vi "储存测试.vi"() -> ()   [LabVIEW 2019, in "test.lvlib"]
uses:
  SubVI/test.lvlib
  <vilib>/Utility/file.llb/Write Delimited Spreadsheet (I64).vi
panel:
  in  "名称或相对路径":string
  out "添加的路径":path
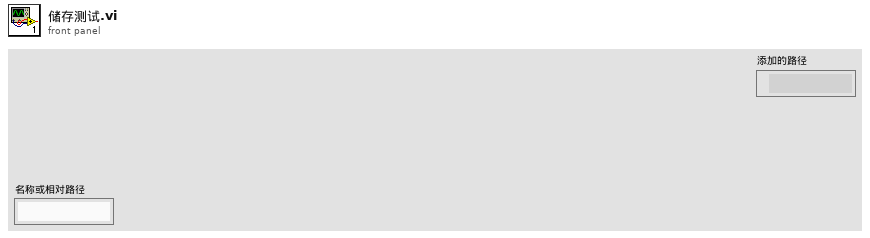
[diagram p1: front panel]
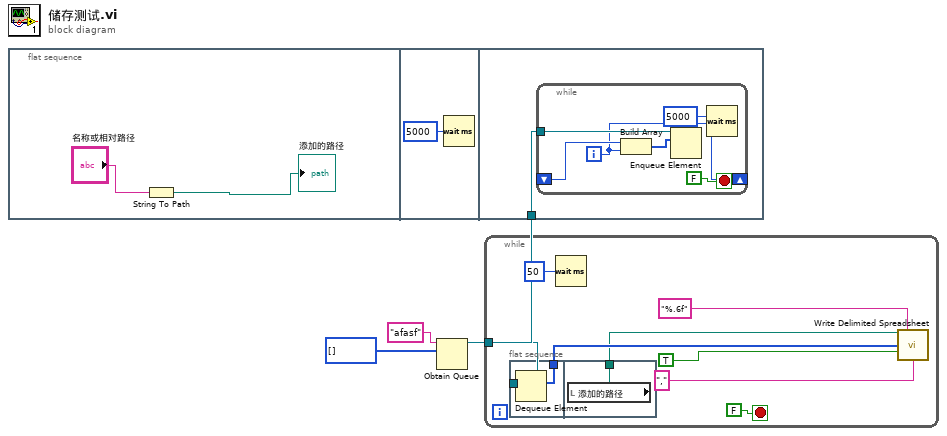
[diagram p0: block diagram]
diagram:
  n1 = flat-sequence {
    tunnel: w1 -> [w7]
    frame #0 {
      n2 = String To Path(string="名称或相对路径") -> (path=→"添加的路径":path)
    }
    frame #1 {
      n3 = Wait (ms)(milliseconds to wait=u32 5000 ("等待时间（毫秒）")) -> ()  [unwired: 1 out]
    }
    frame #2 {
      n4 = while {
        tunnel: w7 -> [w13]
        shift-right: [w11] -> _
        shift-left: _ -> [w12]
        i -> [w11]
        stop <- FALSE stop-if-true
        n5 = Build Array(w12, w11) -> (w10:i32[])
        n6 = Enqueue Element(queue=w13, element=w10) -> ()  [unwired: 2 in, 3 out]
        n7 = Wait (ms)(milliseconds to wait=u32 5000 ("等待时间（毫秒）")) -> ()  [unwired: 1 out]
      }
    }
  }
  n8 = Obtain Queue(name (unnamed)="afasf" ("名称（未命名）"), element data type=i32[] []) -> (queue out=w1:refnum<queue>)  [unwired: 3 in, 2 out]
  n9 = while {
    tunnel: w1 -> [w16]
    stop <- FALSE stop-if-true
    n10 = flat-sequence {
      tunnel: w16 -> [w23]
      tunnel: [w22] -> w15
      tunnel: [w24] -> w14
      frame #0 {
        n11 = Dequeue Element(queue=w23) -> (element=w22:i32[])  [unwired: 2 in, 3 out]
      }
      frame #1 {
        n12 = local read "添加的路径"() -> (w24:path)
      }
    }
    n13 = Wait (ms)(milliseconds to wait=u32 50 ("等待时间（毫秒）")) -> ()  [unwired: 1 out]
    n14 = call-poly <vilib>:"Write Delimited Spreadsheet.vi"("file path (dialog if empty)"=w14, "format (%d)"="%.6f" ("format (%.3f)"), "1D data"=w15, "append to file? (new file:F)"=TRUE, "delimiter (\\t)"="," ("delimiter (\\t)")) -> ()  [unwired: 9 in, 2 out]
  }
